vi "test comm speed.vi"() -> ()   [LabVIEW 2009, in "Magnet.lvclass"]
uses:
  Magnet.lvclass
  Global/Power Supply.vi
panel:
  out "IPSorg":u32
  out "ilm":u32
  out "itc":u32
  out "ips":u32
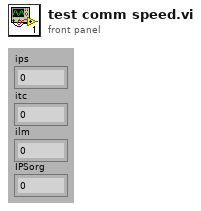
[diagram p1: front panel]
types:
  T1 = typedef "PSIO.ctl" = cluster{"Address":T2, "Version":enum16{"PS", "IPS"}}
  T2 = typedef "OxfordAddress.ctl" = cluster{"Com Port":i32, "ISOBUS Address":i32, "GPIB Address":i16, "Communication":enum16{"RS232", "ISOBUS", "GPIB", "Gateway"}}
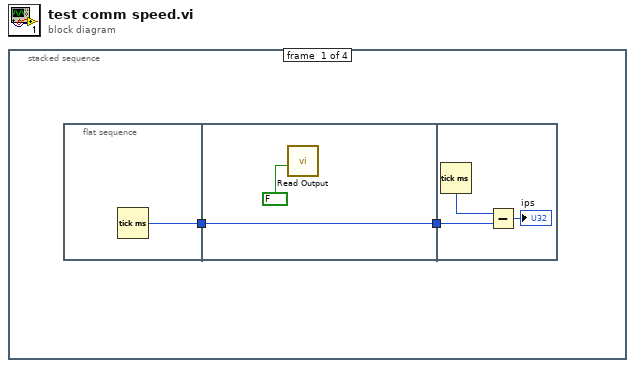
[diagram p0: block diagram]
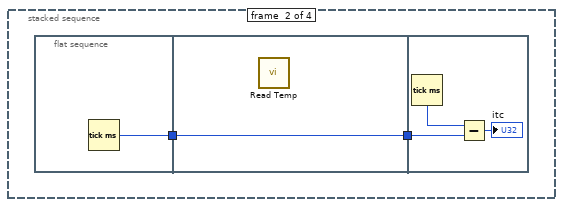
[diagram p2: hidden frame]
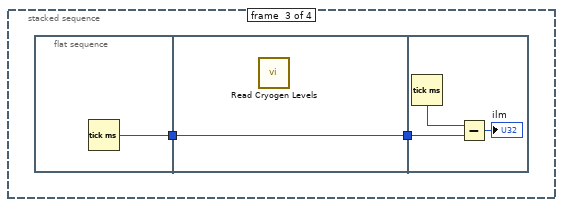
[diagram p3: hidden frame]
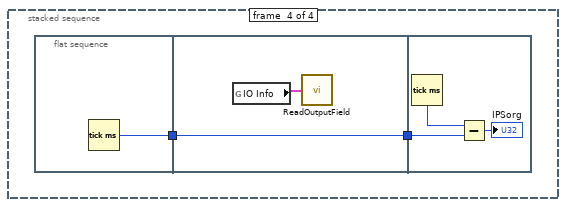
[diagram p4: hidden frame]
diagram:
  n1 = stacked-sequence {
    frame #0 {
      n2 = flat-sequence {
        tunnel: [w3] -> w2
        tunnel: w2 -> [w5]
        tunnel: [w5] -> w1
        tunnel: w1 -> [w7]
        frame #0 {
          n3 = Tick Count (ms)() -> (millisecond timer value=w3:u32)
        }
        frame #1 {
          n4 = call "Read Output.vi"("checkpers?"=FALSE) -> ()  [unwired: 1 in, 6 out]
        }
        frame #2 {
          n5 = Tick Count (ms)() -> (millisecond timer value=w8:u32)
          n6 = Subtract(x=w8, y=w7) -> (x-y=→"ips":u32)
        }
      }
    }
    frame #1 {
      n7 = flat-sequence {
        tunnel: [w11] -> w10
        tunnel: w10 -> [w12]
        tunnel: [w12] -> w9
        tunnel: w9 -> [w14]
        frame #0 {
          n8 = Tick Count (ms)() -> (millisecond timer value=w11:u32)
        }
        frame #1 {
          n9 = call "Read Temp.vi"() -> ()  [unwired: 8 out]
        }
        frame #2 {
          n10 = Tick Count (ms)() -> (millisecond timer value=w15:u32)
          n11 = Subtract(x=w15, y=w14) -> (x-y=→"itc":u32)
        }
      }
    }
    frame #2 {
      n12 = flat-sequence {
        tunnel: [w18] -> w17
        tunnel: w17 -> [w19]
        tunnel: [w19] -> w16
        tunnel: w16 -> [w21]
        frame #0 {
          n13 = Tick Count (ms)() -> (millisecond timer value=w18:u32)
        }
        frame #1 {
          n14 = call "Read Cryogen Levels.vi"() -> ()  [unwired: 12 out]
        }
        frame #2 {
          n15 = Tick Count (ms)() -> (millisecond timer value=w22:u32)
          n16 = Subtract(x=w22, y=w21) -> (x-y=→"ilm":u32)
        }
      }
    }
    frame #3 {
      n17 = flat-sequence {
        tunnel: [w25] -> w24
        tunnel: w24 -> [w27]
        tunnel: [w27] -> w23
        tunnel: w23 -> [w29]
        frame #0 {
          n18 = Tick Count (ms)() -> (millisecond timer value=w25:u32)
        }
        frame #1 {
          n19 = global read "Power Supply.vi" "IO Info"() -> (w26:T1)
          n20 = call "ReadOutputField.vi"("IO Info"=w26) -> ()  [unwired: 3 out]
        }
        frame #2 {
          n21 = Tick Count (ms)() -> (millisecond timer value=w30:u32)
          n22 = Subtract(x=w30, y=w29) -> (x-y=→"IPSorg":u32)
        }
      }
    }
  }
